vi "Blue Stock.vi"   [LabVIEW 2019]
uses:
  Global Var.vi
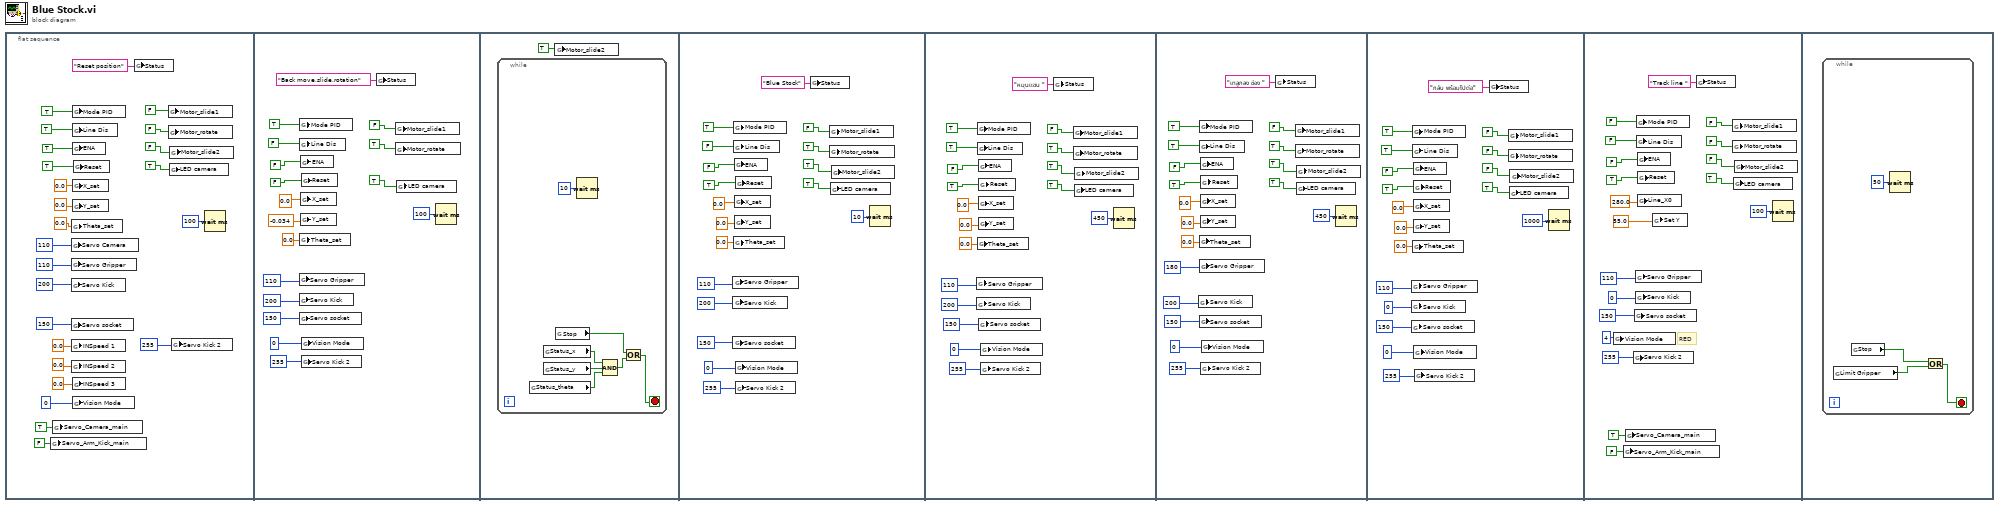
[diagram p0: block diagram]
diagram:
  n1 = flat-sequence {
    frame #0 {
      n2 = global write "Global Var.vi" "Servo_Arm_Kick_main"(FALSE ("Mode PID")) -> ()
      n3 = global write "Global Var.vi" "Servo_Camera_main"(TRUE ("Mode PID")) -> ()
      n4 = global write "Global Var.vi" "Servo Camera"(u8 110 ("Servo Camera")) -> ()
      n5 = global write "Global Var.vi" "Servo Gripper"(u8 110 ("Servo Camera")) -> ()
      n6 = global write "Global Var.vi" "Servo Kick"(u8 200 ("Servo Camera")) -> ()
      n7 = global write "Global Var.vi" "Servo socket"(u8 150 ("Servo Camera")) -> ()
      n8 = global write "Global Var.vi" "Theta_set"(0.0 ("Theta_set")) -> ()
      n9 = global write "Global Var.vi" "INSpeed 1"(0.0 ("X_set")) -> ()
      n10 = global write "Global Var.vi" "INSpeed 2"(0.0 ("Y_set")) -> ()
      n11 = global write "Global Var.vi" "Mode PID"(TRUE ("Mode PID")) -> ()
      n12 = global write "Global Var.vi" "Line Dis"(TRUE ("Mode PID")) -> ()
      n13 = global write "Global Var.vi" "ENA"(TRUE ("ENA")) -> ()
      n14 = global write "Global Var.vi" "X_set"(0.0 ("X_set")) -> ()
      n15 = global write "Global Var.vi" "Y_set"(0.0 ("Y_set")) -> ()
      n16 = global write "Global Var.vi" "INSpeed 3"(0.0 ("Theta_set")) -> ()
      n17 = global write "Global Var.vi" "Vision Mode"(i16 0 ("Vision Mode")) -> ()
      n18 = global write "Global Var.vi" "Reset"(TRUE ("ENA")) -> ()
      n19 = global write "Global Var.vi" "Status"("Reset position" ("Status")) -> ()
      n20 = global write "Global Var.vi" "Motor_slide1"(FALSE ("Mode PID")) -> ()
      n21 = global write "Global Var.vi" "Motor_rotate"(FALSE ("ENA")) -> ()
      n22 = global write "Global Var.vi" "LED camera"(TRUE ("LED camera")) -> ()
      n23 = global write "Global Var.vi" "Motor_slide2"(FALSE ("ENA")) -> ()
      n24 = global write "Global Var.vi" "Servo Kick 2"(u8 255 ("Servo Camera")) -> ()
      n25 = Wait (ms)(milliseconds to wait=u32 100) -> ()  [unwired: 1 out]
    }
    frame #1 {
      n26 = global write "Global Var.vi" "Servo Gripper"(u8 110 ("Servo Camera")) -> ()
      n27 = global write "Global Var.vi" "Servo Kick"(u8 200 ("Servo Camera")) -> ()
      n28 = global write "Global Var.vi" "Servo socket"(u8 150 ("Servo Camera")) -> ()
      n29 = global write "Global Var.vi" "Mode PID"(TRUE ("Mode PID")) -> ()
      n30 = global write "Global Var.vi" "Line Dis"(FALSE ("Mode PID")) -> ()
      n31 = global write "Global Var.vi" "Theta_set"(0.0 ("Theta_set")) -> ()
      n32 = global write "Global Var.vi" "ENA"(FALSE ("ENA")) -> ()
      n33 = global write "Global Var.vi" "X_set"(0.0 ("X_set")) -> ()
      n34 = global write "Global Var.vi" "Y_set"(-0.034 ("Y_set")) -> ()
      n35 = global write "Global Var.vi" "Reset"(FALSE ("ENA")) -> ()
      n36 = global write "Global Var.vi" "Vision Mode"(i16 0 ("Vision Mode")) -> ()
      n37 = global write "Global Var.vi" "Servo Kick 2"(u8 255 ("Servo Camera")) -> ()
      n38 = global write "Global Var.vi" "Status"("Back move,slide,rotation" ("Status")) -> ()
      n39 = global write "Global Var.vi" "Motor_slide1"(FALSE ("Mode PID")) -> ()
      n40 = global write "Global Var.vi" "Motor_rotate"(TRUE ("ENA")) -> ()
      n41 = global write "Global Var.vi" "LED camera"(TRUE ("LED camera")) -> ()
      n42 = Wait (ms)(milliseconds to wait=u32 100) -> ()  [unwired: 1 out]
    }
    frame #2 {
      n43 = while {
        stop <- w45 stop-if-true
        n44 = global read "Global Var.vi" "Status_theta"() -> (w47:bool)
        n45 = global read "Global Var.vi" "Status_x"() -> (w48:bool)
        n46 = global read "Global Var.vi" "Status_y"() -> (w49:bool)
        n47 = global read "Global Var.vi" "Stop"() -> (w43:bool)
        n48 = Wait (ms)(milliseconds to wait=u32 10) -> ()  [unwired: 1 out]
        n49 = Compound Arithmetic op=AND(w48, w49, w47) -> (w44:bool)
        n50 = Or(x=w43, y=w44) -> (x .or. y?=w45:bool)
      }
      n51 = global write "Global Var.vi" "Motor_slide2"(TRUE ("ENA")) -> ()
    }
    frame #3 {
      n52 = global write "Global Var.vi" "Servo Gripper"(u8 110 ("Servo Camera")) -> ()
      n53 = global write "Global Var.vi" "Servo Kick"(u8 200 ("Servo Camera")) -> ()
      n54 = global write "Global Var.vi" "Servo socket"(u8 150 ("Servo Camera")) -> ()
      n55 = global write "Global Var.vi" "Mode PID"(TRUE ("Mode PID")) -> ()
      n56 = global write "Global Var.vi" "Line Dis"(FALSE ("Mode PID")) -> ()
      n57 = global write "Global Var.vi" "Theta_set"(0.0 ("Theta_set")) -> ()
      n58 = global write "Global Var.vi" "ENA"(FALSE ("ENA")) -> ()
      n59 = global write "Global Var.vi" "X_set"(0.0 ("X_set")) -> ()
      n60 = global write "Global Var.vi" "Y_set"(0.0 ("Y_set")) -> ()
      n61 = global write "Global Var.vi" "Reset"(TRUE ("ENA")) -> ()
      n62 = global write "Global Var.vi" "Vision Mode"(i16 0 ("Vision Mode")) -> ()
      n63 = global write "Global Var.vi" "Servo Kick 2"(u8 255 ("Servo Camera")) -> ()
      n64 = global write "Global Var.vi" "Status"("Blue Stock" ("Status")) -> ()
      n65 = global write "Global Var.vi" "Motor_slide1"(FALSE ("Mode PID")) -> ()
      n66 = global write "Global Var.vi" "Motor_rotate"(TRUE ("ENA")) -> ()
      n67 = global write "Global Var.vi" "LED camera"(TRUE ("LED camera")) -> ()
      n68 = global write "Global Var.vi" "Motor_slide2"(TRUE ("ENA")) -> ()
      n69 = Wait (ms)(milliseconds to wait=u32 10) -> ()  [unwired: 1 out]
    }
    frame #4 {
      n70 = global write "Global Var.vi" "Servo Gripper"(u8 110 ("Servo Camera")) -> ()
      n71 = global write "Global Var.vi" "Servo Kick"(u8 200 ("Servo Camera")) -> ()
      n72 = global write "Global Var.vi" "Mode PID"(TRUE ("Mode PID")) -> ()
      n73 = global write "Global Var.vi" "Line Dis"(TRUE ("Mode PID")) -> ()
      n74 = global write "Global Var.vi" "Theta_set"(0.0 ("Theta_set")) -> ()
      n75 = global write "Global Var.vi" "ENA"(FALSE ("ENA")) -> ()
      n76 = global write "Global Var.vi" "X_set"(0.0 ("X_set")) -> ()
      n77 = global write "Global Var.vi" "Y_set"(0.0 ("Y_set")) -> ()
      n78 = global write "Global Var.vi" "Reset"(TRUE ("ENA")) -> ()
      n79 = global write "Global Var.vi" "Servo socket"(u8 150 ("Servo Camera")) -> ()
      n80 = global write "Global Var.vi" "Vision Mode"(i16 0 ("Vision Mode")) -> ()
      n81 = global write "Global Var.vi" "Servo Kick 2"(u8 255 ("Servo Camera")) -> ()
      n82 = global write "Global Var.vi" "Status"("หมุนเเขน " ("Status")) -> ()
      n83 = global write "Global Var.vi" "Motor_slide1"(FALSE ("Mode PID")) -> ()
      n84 = global write "Global Var.vi" "Motor_rotate"(TRUE ("ENA")) -> ()
      n85 = global write "Global Var.vi" "LED camera"(TRUE ("LED camera")) -> ()
      n86 = global write "Global Var.vi" "Motor_slide2"(TRUE ("ENA")) -> ()
      n87 = Wait (ms)(milliseconds to wait=u32 450) -> ()  [unwired: 1 out]
    }
    frame #5 {
      n88 = global write "Global Var.vi" "Servo Kick"(u8 200 ("Servo Camera")) -> ()
      n89 = global write "Global Var.vi" "Mode PID"(TRUE ("Mode PID")) -> ()
      n90 = global write "Global Var.vi" "Line Dis"(TRUE ("Mode PID")) -> ()
      n91 = global write "Global Var.vi" "Theta_set"(0.0 ("Theta_set")) -> ()
      n92 = global write "Global Var.vi" "Servo Gripper"(u8 180 ("Servo Camera")) -> ()
      n93 = global write "Global Var.vi" "Servo socket"(u8 150 ("Servo Camera")) -> ()
      n94 = global write "Global Var.vi" "ENA"(FALSE ("ENA")) -> ()
      n95 = global write "Global Var.vi" "X_set"(0.0 ("X_set")) -> ()
      n96 = global write "Global Var.vi" "Y_set"(0.0 ("Y_set")) -> ()
      n97 = global write "Global Var.vi" "Reset"(TRUE ("ENA")) -> ()
      n98 = global write "Global Var.vi" "Servo Kick 2"(u8 255 ("Servo Camera")) -> ()
      n99 = global write "Global Var.vi" "Vision Mode"(i16 0 ("Vision Mode")) -> ()
      n100 = global write "Global Var.vi" "Status"("เทลูกลง ช่อง " ("Status")) -> ()
      n101 = global write "Global Var.vi" "Motor_slide1"(FALSE ("Mode PID")) -> ()
      n102 = global write "Global Var.vi" "Motor_rotate"(TRUE ("ENA")) -> ()
      n103 = global write "Global Var.vi" "LED camera"(TRUE ("LED camera")) -> ()
      n104 = global write "Global Var.vi" "Motor_slide2"(TRUE ("ENA")) -> ()
      n105 = Wait (ms)(milliseconds to wait=u32 450) -> ()  [unwired: 1 out]
    }
    frame #6 {
      n106 = global write "Global Var.vi" "Servo Gripper"(u8 110 ("Servo Camera")) -> ()
      n107 = global write "Global Var.vi" "Servo Kick"(u8 0 ("Servo Camera")) -> ()
      n108 = global write "Global Var.vi" "Servo socket"(u8 150 ("Servo Camera")) -> ()
      n109 = global write "Global Var.vi" "Mode PID"(TRUE ("Mode PID")) -> ()
      n110 = global write "Global Var.vi" "Line Dis"(TRUE ("Mode PID")) -> ()
      n111 = global write "Global Var.vi" "Theta_set"(0.0 ("Theta_set")) -> ()
      n112 = global write "Global Var.vi" "ENA"(FALSE ("ENA")) -> ()
      n113 = global write "Global Var.vi" "X_set"(0.0 ("X_set")) -> ()
      n114 = global write "Global Var.vi" "Y_set"(0.0 ("Y_set")) -> ()
      n115 = global write "Global Var.vi" "Reset"(TRUE ("ENA")) -> ()
      n116 = global write "Global Var.vi" "Vision Mode"(i16 0 ("Vision Mode")) -> ()
      n117 = global write "Global Var.vi" "Servo Kick 2"(u8 255 ("Servo Camera")) -> ()
      n118 = global write "Global Var.vi" "Status"("กลับ พร้อมไปต่อ" ("Status")) -> ()
      n119 = global write "Global Var.vi" "Motor_slide1"(FALSE ("Mode PID")) -> ()
      n120 = global write "Global Var.vi" "Motor_rotate"(FALSE ("ENA")) -> ()
      n121 = global write "Global Var.vi" "LED camera"(TRUE ("LED camera")) -> ()
      n122 = global write "Global Var.vi" "Motor_slide2"(FALSE ("ENA")) -> ()
      n123 = Wait (ms)(milliseconds to wait=u32 1000) -> ()  [unwired: 1 out]
    }
    frame #7 {
      # "RED"
      n124 = global write "Global Var.vi" "Vision Mode"(i16 4 ("Vision Mode")) -> ()
      n125 = global write "Global Var.vi" "Servo_Arm_Kick_main"(FALSE ("Mode PID")) -> ()
      n126 = global write "Global Var.vi" "Servo_Camera_main"(TRUE ("Mode PID")) -> ()
      n127 = global write "Global Var.vi" "Servo Kick 2"(u8 255 ("Servo Camera")) -> ()
      n128 = global write "Global Var.vi" "Servo socket"(u8 150 ("Servo Camera")) -> ()
      n129 = global write "Global Var.vi" "Servo Gripper"(u8 110 ("Servo Camera")) -> ()
      n130 = global write "Global Var.vi" "Servo Kick"(u8 0 ("Servo Camera")) -> ()
      n131 = global write "Global Var.vi" "Mode PID"(FALSE ("Mode PID")) -> ()
      n132 = global write "Global Var.vi" "Line Dis"(FALSE ("Mode PID")) -> ()
      n133 = global write "Global Var.vi" "ENA"(FALSE ("ENA")) -> ()
      n134 = global write "Global Var.vi" "Line_X0"(280.0 ("Y_set")) -> ()
      n135 = global write "Global Var.vi" "Reset"(TRUE ("ENA")) -> ()
      n136 = global write "Global Var.vi" "Set Y"(55.0 ("Y_set")) -> ()
      n137 = global write "Global Var.vi" "Status"("Track line " ("Status")) -> ()
      n138 = global write "Global Var.vi" "Motor_slide1"(FALSE ("Mode PID")) -> ()
      n139 = global write "Global Var.vi" "Motor_rotate"(FALSE ("ENA")) -> ()
      n140 = global write "Global Var.vi" "LED camera"(TRUE ("LED camera")) -> ()
      n141 = global write "Global Var.vi" "Motor_slide2"(FALSE ("ENA")) -> ()
      n142 = Wait (ms)(milliseconds to wait=u32 100) -> ()  [unwired: 1 out]
    }
    frame #8 {
      n143 = while {
        stop <- w143 stop-if-true
        n144 = global read "Global Var.vi" "Limit Gripper"() -> (w141:bool)
        n145 = global read "Global Var.vi" "Stop"() -> (w142:bool)
        n146 = Wait (ms)(milliseconds to wait=u32 50) -> ()  [unwired: 1 out]
        n147 = Or(x=w142, y=w141) -> (x .or. y?=w143:bool)
      }
    }
  }
